vi "sub_DTMF_Format Rx Data.vi"(0 "DTMF Settings":T1={"My Phone Number"="", "Ring Tone"=FALSE, "Quantization Level"=4, "\nGray Encoding"=FALSE} {"Quantization Level" items=["2"=2, "4"=4, "8"=8, "16"=16]}, 2 "Ringtone Path":path=path "C:/Users/Sungeun/Dropbox/Lab/DTMF/VI Source/Project 3/ringtone/Nokia_Original.wav", 4 "Output Packet Array":i32[][](array[numeric])) -> (3 "dequants":dbl[](array[numeric]), 5 "Received Message":string, 6 "Received Digits":string)   [LabVIEW 2011]
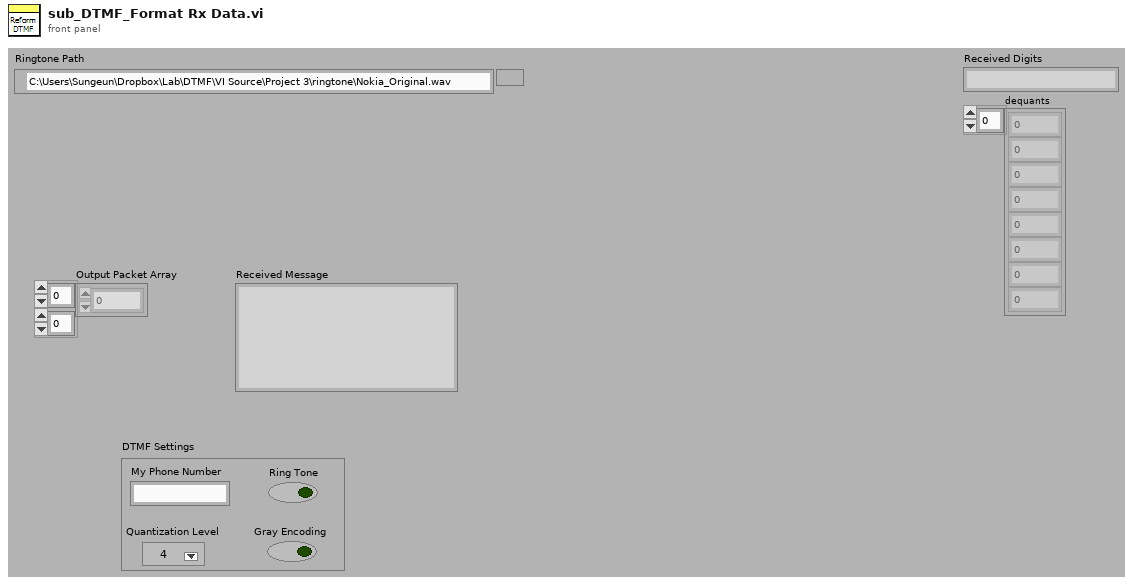
[diagram p1: front panel]
types:
  T1 = cluster{"My Phone Number":string, "Ring Tone":bool, "Quantization Level":u16, "\nGray Encoding":bool}
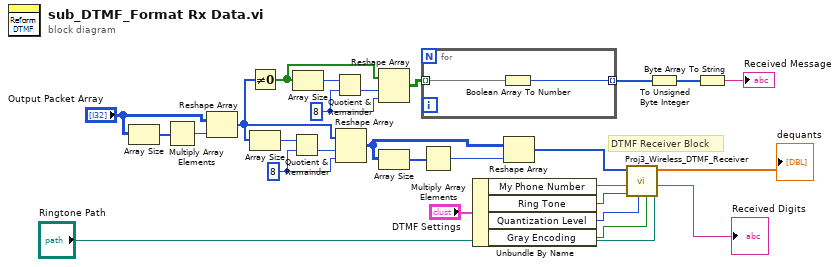
[diagram p0: block diagram]
diagram:
  w16 = 8 ("dimension size")
  w25 = 8 ("dimension size")
  # "DTMF Receiver Block"
  n1 = Array Size(array="Output Packet Array") -> (size(s)=w20:i32[])
  n2 = Multiply Array Elements(1:w20) -> (0:w22:i32)
  n3 = Reshape Array("Output Packet Array", w22) -> (w13:i32[])
  n4 = Not Equal To 0?(x=w13) -> (x != 0?=w23:bool[])
  n5 = Array Size(array=w13) -> (size(s)=w15:i32)
  n6 = Quotient & Remainder(x=w15, y=w16) -> (floor(x/y)=w14:i32)  [unwired: 1 out]
  n7 = Array Size(array=w23) -> (size(s)=w24:i32)
  n8 = Quotient & Remainder(x=w24, y=w25) -> (floor(x/y)=w19:i32)  [unwired: 1 out]
  n9 = Reshape Array(w13, w14, w16) -> (w10:i32[][])
  n10 = Reshape Array(w23, w19, w25) -> (w17:bool[][])
  n11 = Array Size(array=w10) -> (size(s)=w11:i32[])
  n12 = for {
    tunnel: w17 -> [w29] mode=indexing
    tunnel: [w28] -> w26 mode=indexing
    n13 = Boolean Array To Number(Boolean array=w29) -> (number=w28:u32)
  }
  n14 = Multiply Array Elements(1:w11) -> (0:w12:i32)
  n15 = Unbundle By Name("DTMF Settings") -> ("My Phone Number"=w3:string, "Ring Tone"=w4:bool, "Quantization Level"=w6:u16, "Gray Encoding"=w5:bool)
  n16 = Reshape Array(w10, w12) -> (w9:i32[])
  n17 = call "Proj3_Wireless_DTMF_Receiver.vi"("Ringtone Path"="Ringtone Path", "Gray Bit Encoding"=w5, "Quantization Level"=w6, "Ringtone"=w4, "My Phone Number"=w3, "RXbitStream"=w9) -> ("Received Digits"=→"Received Digits":string, "dequants"=→"dequants":dbl[])  [unwired: 4 in]
  n18 = To Unsigned Byte Integer(number=w26) -> (unsigned 8bit integer=w18:u8[])
  n19 = Byte Array To String(unsigned byte array=w18) -> (string=→"Received Message":string)
